vi "HEWH Gas Thermal Raw Calc.vi"(1 "Use Constant Thermal Efficiency":bool, 5 "RTD Out (Deg F)":dbl, 7 "Constant Thermal Eff":dbl format="%#.5g", 9 "RTD In (Deg F)":dbl, 11 "error in (no error)":errorcluster, 12 "Gallons (Gal)":dbl) -> (4 "Rate":dbl, 6 "Eff":dbl format="%#.5g", 15 "error out":errorcluster)   [LabVIEW 2023]
uses:
  Macros/UEF/Type Definitions/HEWH Water Properties.ctl
  Utility/Type Definitions/UTILITY Notifier.ctl
panel:
  out "B":dbl
  out "A":dbl
  out "Heat input":dbl
  # "Common Parameters"
  # "Real Time Calculation of Thermal (False)"
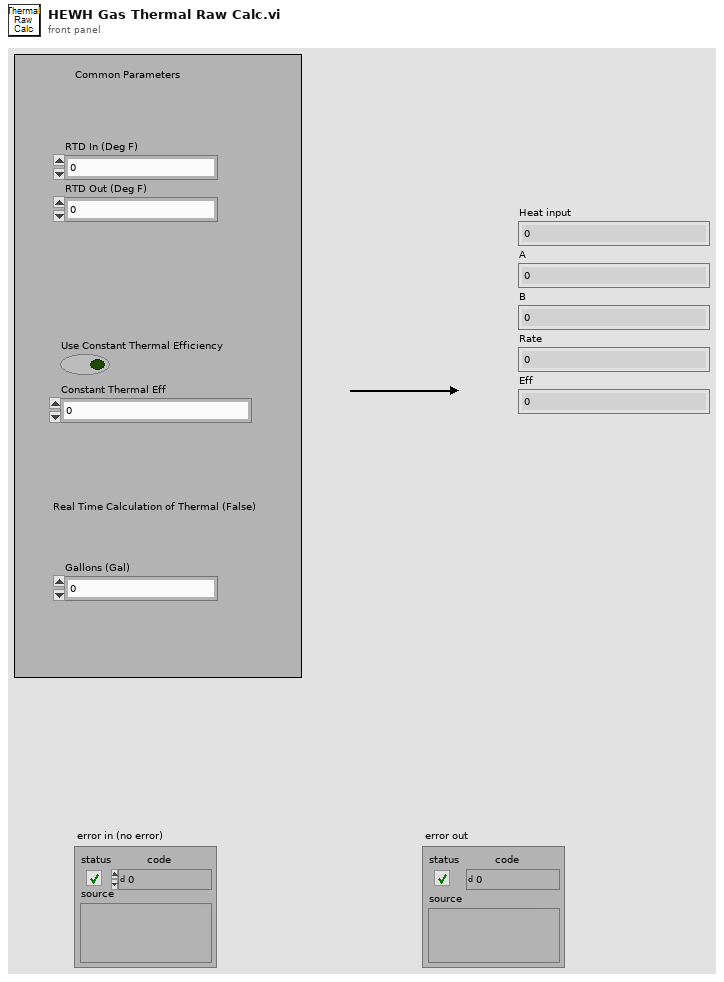
[diagram p1: front panel]
types:
  T1 = typedef "UTILITY Notifier.ctl" = enum16{"Set", "Read", "Release Ref"}
  T2 = typedef "HEWH Water Properties.ctl" = enum16{"GEA Intertek Values", "CSA Values", "ANSI Values"}
  T3 = typedef "Inficon Data.ctl" = cluster{"Gross Heating Value, Vol (Real, Dry)":dbl, "Nitrogen Component Normalized Mole % (Dry)":dbl, "Methane Component Normalized Mole % (Dry)":dbl, "Carbon Dioxide Component Normalized Mole % (Dry)":dbl, "Ethane Component Normalized Mole % (Dry)":dbl, "Propane Component Normalized Mole % (Dry)":dbl, "i-Pentane Component Normalized Mole % (Dry)":dbl, "i-Butane Component Normalized Mole % (Dry)":dbl, "n-Butane Component Normalized Mole % (Dry)":dbl, "n-Pentane Component Normalized Mole % (Dry)":dbl, "Hexane Component Normalized Mole % (Dry)":dbl, "Heptane Component Normalized Mole % (Dry)":dbl, "Gross Wobbe Index, Real(Dry)":dbl, "Relative Density, Real(Dry)":dbl, "Propylene Component Normalized Mole % (Dry)":dbl, "C4 Olefins Component Normalized Mole % (Dry)":dbl, "Water Component Normalized Mole % (Dry)":dbl, "Gross Heating Value, Vol (Real, Sat)":dbl, "Natural Gas Data":string[][], "Propane Data":string[][]}
  T4 = typedef "Data Cluster.ctl" = cluster{"Absolute Pressure":dbl, "Gauge/Diff. Pressure":dbl, "Barometric Pressure":dbl, "Temperature":dbl, "Volumetric Flow":dbl, "Mass Flow":dbl, "Setpoint":dbl, "Valve Drive":dbl, "Totalizer":dbl, "[hr]":dbl, "[min]":dbl, "[sec]":dbl, "Totalizer Average Flow":dbl, "Totalizer Peak Flow":dbl, "Gas selected":string}
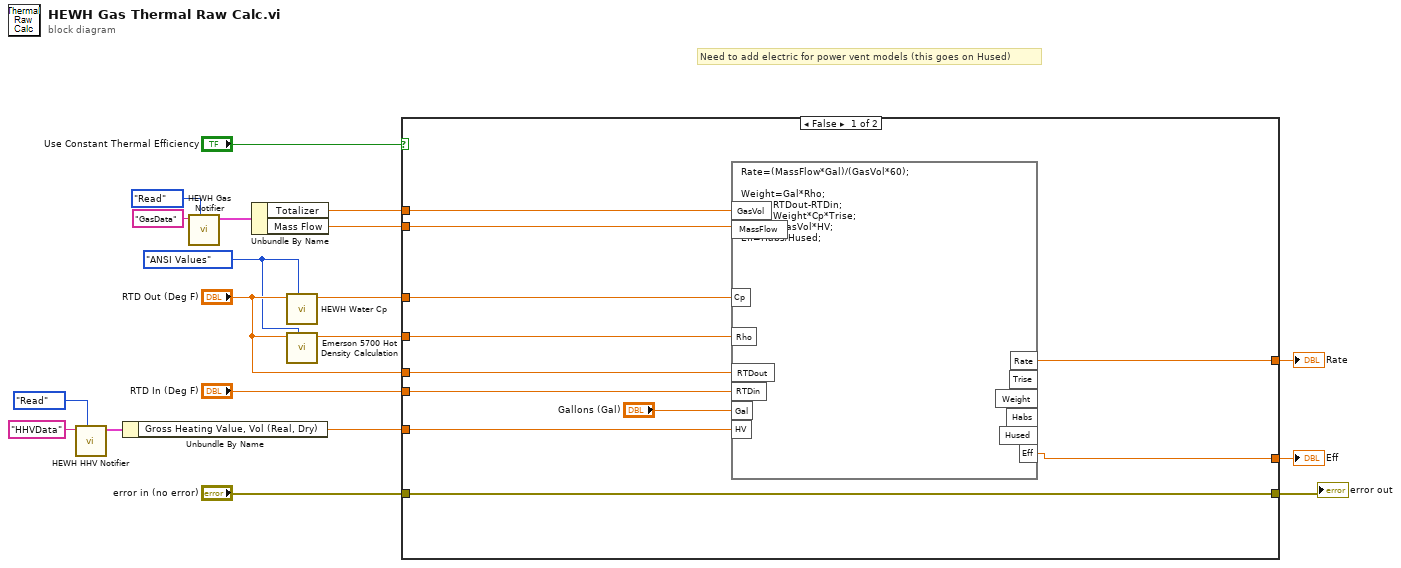
[diagram p0: block diagram]
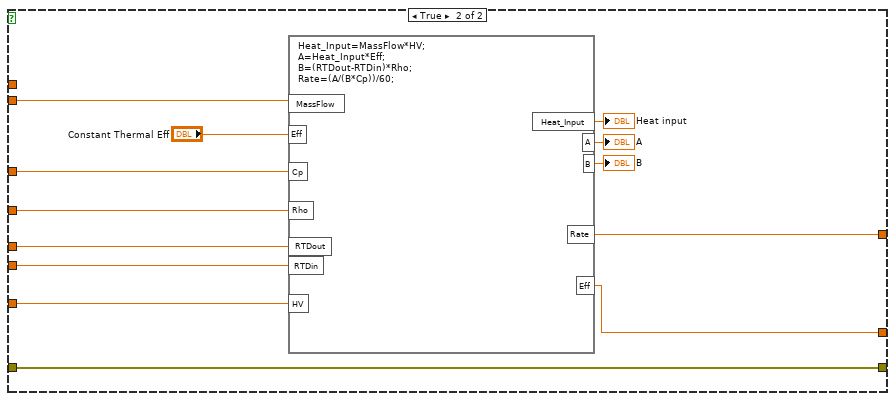
[diagram p2: hidden frame]
diagram:
  w13 = HEWH_Water_Properties."ANSI Values" ("Water Properties Reference")
  # "Need to add electric for power vent models (this goes on Hused)"
  n1 = call "HEWH HHV Notifier.vi"("Status"=UTILITY_Notifier."Read", "name (unnamed)"="HHVData") -> ("Gas Measurment Data Output"=w2:T3)  [unwired: 8 in, 1 out]
  n2 = Unbundle By Name(w2) -> ("Gross Heating Value, Vol (Real, Dry)"=w1:dbl)
  n3 = call "HEWH Gas Notifier.vi"("Status"=UTILITY_Notifier."Read", "name (unnamed)"="GasData") -> ("Gas Measurment Data Output"=w9:T4)  [unwired: 8 in, 1 out]
  n4 = Unbundle By Name(w9) -> ("Totalizer"=w5:dbl, "Mass Flow"=w6:dbl)
  n5 = call "HEWH Water Cp.vi"("Water Properties Reference"=w13, "Input Temperature (°F)"="RTD Out (Deg F)") -> ("Specific Heat (BTU/lbm*F)"=w14:dbl)  [unwired: 8 in, 1 out]
  n6 = call "Emerson 5700 Hot Density Calculation.vi"("Water Properties Reference"=w13, "RTD Out (°F)"="RTD Out (Deg F)") -> ("Density (lb/gal)"=w15:dbl)  [unwired: 8 in, 1 out]
  n7 = case shown="False" "Use Constant Thermal Efficiency" {
    tunnel: [w29 w43] -> w19
    tunnel: "error in (no error)" -> [w29 w43]
    tunnel: "RTD Out (Deg F)" -> [w28 w41]
    tunnel: w15 -> [w27 w37]
    tunnel: w14 -> [w26 w38]
    tunnel: "RTD In (Deg F)" -> [w25 w42]
    tunnel: w1 -> [w24 w40]
    tunnel: w6 -> [w23 w39]
    tunnel: [w22 w35] -> w11
    tunnel: [w21 w31] -> w10
    tunnel: w5 -> [w20 _]
    frame False {
      n8 = formula code="Rate=(MassFlow*Gal)/(GasVol*60);\n\nWeight=Gal*Rho;\nTrise=RTDout-RTDin;\nHabs=Weight*Cp*Trise;\nHused=GasVol*HV;\nEff=Habs/Hused;"("RTDout"=w28, "RTDin"=w25, "MassFlow"=w23, "Gal"="Gallons (Gal)", "GasVol"=w20, "HV"=w24, "Cp"=w26, "Rho"=w27) -> ("Rate"=w22:dbl, "Eff"=w21:dbl)  [unwired: 4 out]
    }
    frame True {
      n9 = formula code="Heat_Input=MassFlow*HV;\nA=Heat_Input*Eff;\nB=(RTDout-RTDin)*Rho;\nRate=(A/(B*Cp))/60;"("RTDout"=w41, "RTDin"=w42, "MassFlow"=w39, "HV"=w40, "Cp"=w38, "Rho"=w37, "Eff"="Constant Thermal Eff") -> ("Rate"=w35:dbl, "Heat_Input"=→"Heat input":dbl, "A"=→"A":dbl, "B"=→"B":dbl, "Eff"=w31:dbl)
    }
  }
  "error out" <- w19
  "Rate" <- w11
  "Eff" <- w10
